vi "Create All Message Queues.vi"(8 "error in (no error)":errorcluster, 10 "Master Queue In":refnum<queue>, 11 "Stand alone?":bool) -> (0 "error out":errorcluster, 3 "Message Queues out":T1)   [LabVIEW 2013, in "AvaSpec Message Queue.lvlib"]
doc: "This VI creates and initializes all the message queues for your application. If your application requires more than one message queue, right-click the \"Message Queues\" constant above and select Open Type Def. Add the new Message Queue(s) to the type definition, then initialize them in this VI."
uses:
  AvaSpec Message Queue.lvlib
  All Message Queues.ctl
  Message Cluster.ctl
  Enqueue Message (Single).vi
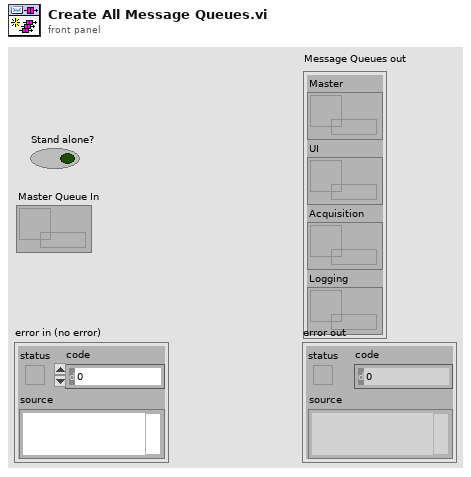
[diagram p1: front panel]
types:
  T1 = typedef "AvaSpec Message Queue.lvlib/All Message Queues.ctl" = cluster{"Master":refnum<queue>, "UI":refnum<queue>, "Acquisition":refnum<queue>, "Logging":refnum<queue>}
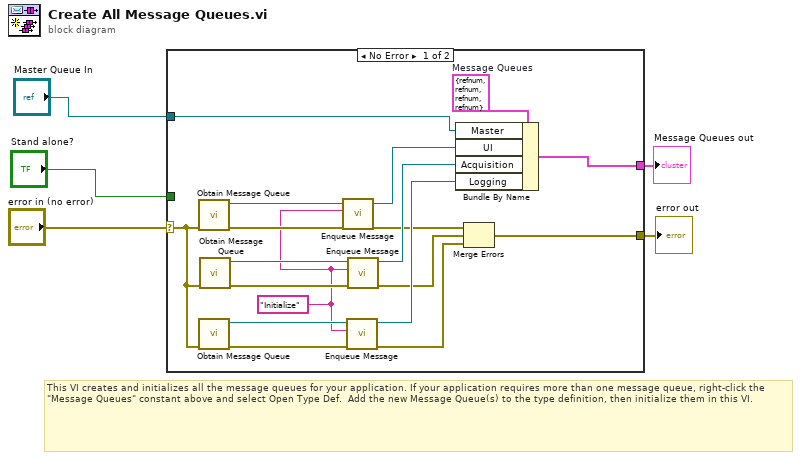
[diagram p0: block diagram]
diagram:
  # "This VI creates and initializes all the message queues for your application. If your application requires more than one message queue, right-click the \"Message Queues\" constant above and select Open Type Def.  Add the new Message Queue(s) to the type definition, then initialize them in this VI."
  n1 = case shown="No Error" "error in (no error)" {
    selector: "error in (no error)" -> [w16 w23]
    tunnel: [w13 w23] -> w5
    tunnel: [w21 _] -> w4
    tunnel: "Stand alone?" -> [_ _]
    tunnel: "Master Queue In" -> [w6 _]
    frame No Error {
      w8 = "Initialize" ("Message")
      w22 = T1 {"Master"=refnum, "UI"=refnum, "Acquisition"=refnum, "Logging"=refnum}  # Message Queues
      n2 = call "Obtain Message Queue.vi"("error in (no error)"=w16) -> ("error out"=w9:errorcluster, "Message Queue"=w7:refnum<queue>)  [unwired: 9 in]
      n3 = call "Obtain Message Queue.vi"("error in (no error)"=w16) -> ("error out"=w18:errorcluster, "Message Queue"=w17:refnum<queue>)  [unwired: 9 in]
      n4 = call "Obtain Message Queue.vi"("error in (no error)"=w16) -> ("error out"=w19:errorcluster, "Message Queue"=w20:refnum<queue>)  [unwired: 9 in]
      n5 = call-poly "Enqueue Message.vi"("Message"=w8, "Message Queue"=w7) -> ("dup Message Queue"=w10:refnum<queue>)  [unwired: 8 in, 1 out]
      n6 = call-poly "Enqueue Message.vi"("error in (no error)"=w18, "Message"=w8, "Message Queue"=w17) -> ("error out"=w11:errorcluster, "dup Message Queue"=w14:refnum<queue>)  [unwired: 7 in]
      n7 = call-poly "Enqueue Message.vi"("error in (no error)"=w19, "Message"=w8, "Message Queue"=w20) -> ("error out"=w12:errorcluster, "dup Message Queue"=w15:refnum<queue>)  [unwired: 7 in]
      n8 = Bundle By Name(cluster=w22, "Master"=w6, "UI"=w10, "Acquisition"=w15, "Logging"=w14) -> (w21:T1)
      n9 = Merge Errors(w9, w12, w11) -> (w13:errorcluster)
    }
    frame Error {
    }
  }
  "Message Queues out" <- w4
  "error out" <- w5
